vi "Uncaging UI.vi"() -> ()   [LabVIEW 2012]
uses:
  <vilib>/vision/Image Controls.llb/IMAQ Image.ctl
  GFG/GFG Translator Wrapper/GFGTranslator_Action.ctl
  GFG/GFG Translator Wrapper/GFGTranslator_Datatype.ctl
panel:
  in  "Grab SciScan Image":bool
  in  "stop uncaging UI":bool
  out "Image":T1(plugin-control)
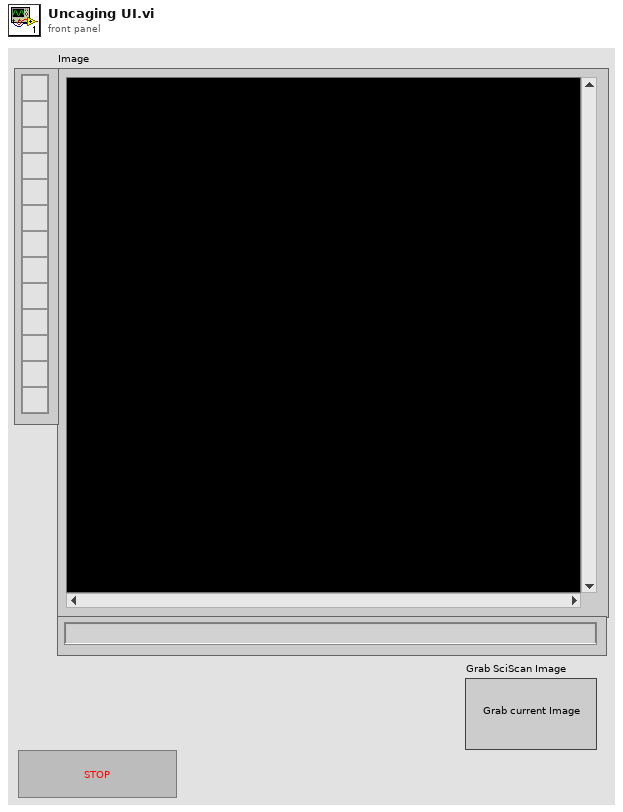
[diagram p1: front panel]
types:
  T1 = typedef "IMAQ Image.ctl" = refnum<image>
  T2 = typedef "GFGTranslator_Datatype.ctl" = enum16{"String", "Path (String)", "Numeric", "Boolean", "Set_BoolRef (use boolean data)", "Get_Variant", "Get_2DArray (I16)", "Get_Image_2DArray (I16)", "Get_Version (String)", "Get_All GFG variables (String)"}
  T3 = typedef "GFGTranslator_Action.ctl" = enum16{"Get", "Set"}
  T4 = typedef "GFGTranslator_errors.ctl" = enum16{"Success", "SciScan Not Running", "No Get Method for Selected Datatype", "No Set Method for Selected Datatype", "Variable Not Found", "Unexpected Datatype"}
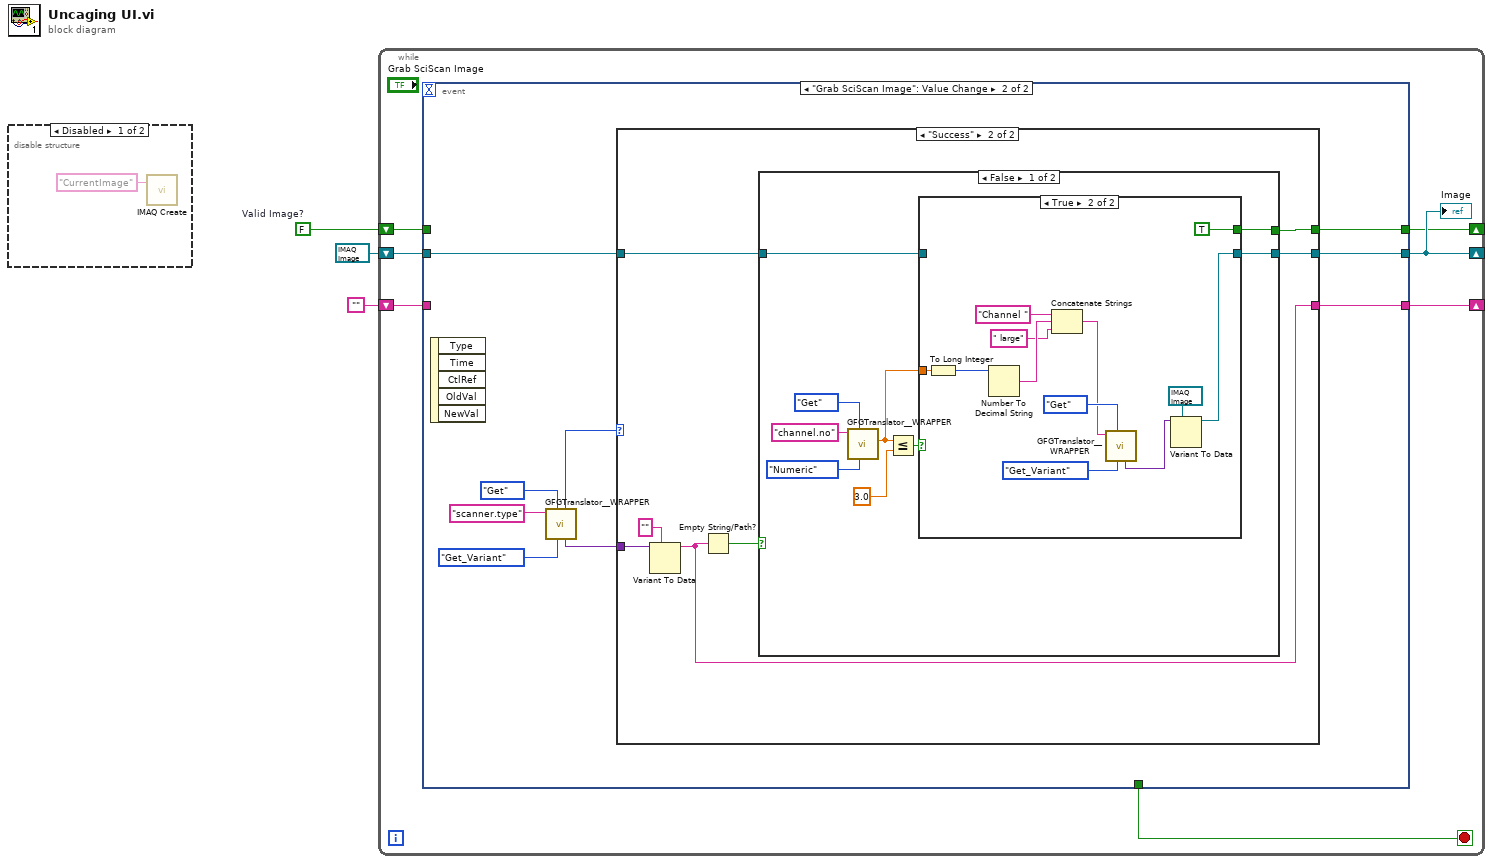
[diagram p0: block diagram]
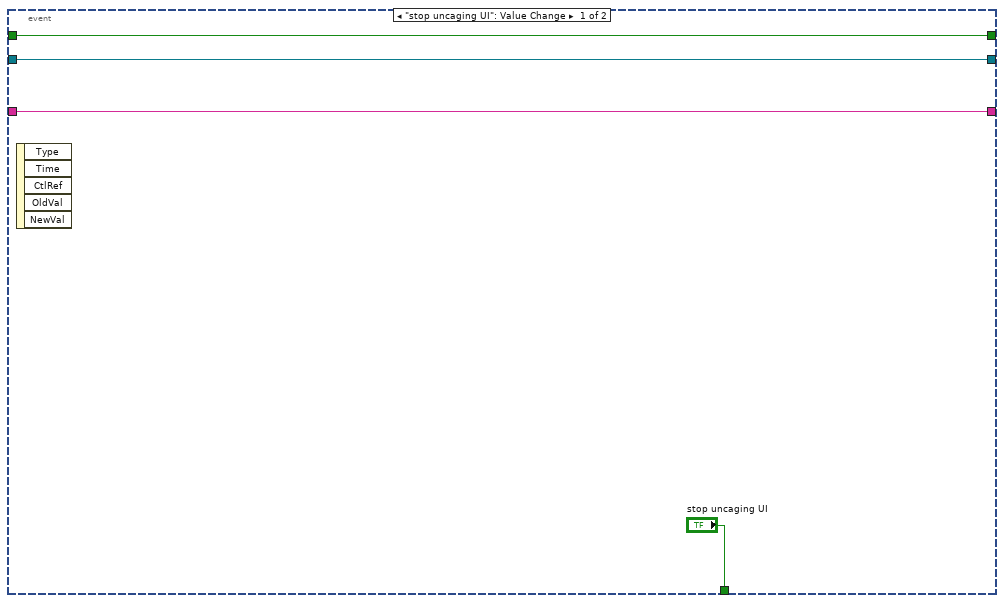
[diagram p3: hidden frame]
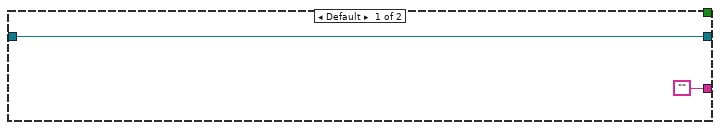
[diagram p4: hidden frame]
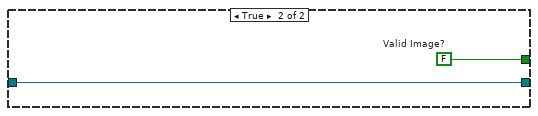
[diagram p6: hidden frame]
diagram:
  w3 = FALSE  # Valid Image?
  n1 = disable-structure shown="Disabled" {
    frame Disabled {
      n2 = call "IMAQ Create"("Image Name"="CurrentImage") -> ()  [unwired: 4 in, 2 out]
    }
    frame Enabled {
    }
  }
  n3 = while {
    shift-right: [w5] -> _
    shift-left: "" -> [w10]
    shift-right: [w6] -> _
    shift-left: w3 -> [w8]
    shift-right: [w7] -> _
    shift-left: T1 refnum ("Image") -> [w9]
    stop <- w11 stop-if-true
    n4 = event shown="[1] \"Grab SciScan Image\": Value Change" {
      selector: _ -> [_ _]
      dyn-events: _ -> [_ _]
      timeout: _ -> [_ _]
      tunnel: ["stop uncaging UI" _] -> w11
      tunnel: w10 -> [w12 _]
      tunnel: w9 -> [w14 w21]
      tunnel: w8 -> [w13 _]
      tunnel: [w14 w20] -> w7
      tunnel: [w13 w19] -> w6
      tunnel: [w12 w17] -> w5
      event "stop uncaging UI": Value Change {
        n5 = event-data() -> ()  [unwired: 1 in, 5 out]
      }
      event "Grab SciScan Image": Value Change {
        n6 = event-data() -> ()  [unwired: 1 in, 5 out]
        n7 = call "GFGTranslator__WRAPPER.vi"("GFGTranslator Datatype"=GFGTranslator_Datatype."Get_Variant", "GFG Translator Action"=GFGTranslator_Action."Get", "GFG Variable Name"="scanner.type" ("Variable Name in")) -> ("Variant_Output"=w16:variant, "Status Output"=w18:T4)  [unwired: 3 in, 4 out]
        n8 = case shown="\"Success\"" w18 {
          tunnel: w21 -> [w26 w33]
          tunnel: [w26 w32] -> w20
          tunnel: [_ w31] -> w19
          tunnel: ["" w28] -> w17
          tunnel: w16 -> [_ w30]
          frame Default {
          }
          frame "Success" {
            n9 = Variant To Data(type="" ("GFG Variable Name"), Variant=w30) -> (data=w28:string)  [unwired: 1 in, 1 out]
            n10 = Empty String/Path?(string/path=w28) -> (empty?=w27:bool)
            n11 = case shown="False" w27 {
              tunnel: w33 -> [w36 w57]
              tunnel: [w35 w57] -> w32
              tunnel: [w34 w56] -> w31
              frame False {
                n12 = call "GFGTranslator__WRAPPER.vi"("GFGTranslator Datatype"=GFGTranslator_Datatype."Numeric", "GFG Translator Action"=GFGTranslator_Action."Get", "GFG Variable Name"="channel.no") -> ("Numeric_Output"=w37:dbl)  [unwired: 3 in, 5 out]
                n13 = Less Or Equal?(x=w37, y=3.0) -> (x <= y?=w38:bool)
                n14 = case shown="True" w38 {
                  tunnel: w37 -> [_ w50]
                  tunnel: w36 -> [w43 _]
                  tunnel: [w43 w46] -> w35
                  tunnel: [_ TRUE ("Valid Image?")] -> w34
                  frame False {
                  }
                  frame True {
                    n15 = To Long Integer(number=w50) -> (32bit integer=w44:i32)
                    n16 = Number To Decimal String(number=w44) -> (decimal integer string=w52:string)  [unwired: 1 in]
                    n17 = Concatenate Strings("Channel " ("GFG Variable Name"), w52, " large" ("string")) -> (w47:string)
                    n18 = call "GFGTranslator__WRAPPER.vi"("GFGTranslator Datatype"=GFGTranslator_Datatype."Get_Variant", "GFG Translator Action"=GFGTranslator_Action."Get", "GFG Variable Name"=w47) -> ("Variant_Output"=w48:variant)  [unwired: 3 in, 5 out]
                    n19 = Variant To Data(type=T1 refnum ("Image"), Variant=w48) -> (data=w46:T1)  [unwired: 1 in, 1 out]
                  }
                }
              }
              frame True {
                w56 = FALSE  # Valid Image?
              }
            }
          }
        }
      }
    }
    "Image" <- w7
  }
